vi "Lookup Group.vi"(7 "Group Type (Abstract)":refnum<class "GroupAbstract.lvclass">, 8 "error in (no error)":errorcluster, 10 "Group Name":string, 11 "Module in":refnum<class "Module.lvclass">) -> (0 "error out":errorcluster, 2 "Group":refnum<class "GroupAbstract.lvclass">, 3 "Module out":refnum<class "Module.lvclass">)   [LabVIEW 2020, in "Volatus.lvlib" / "Module.lvclass"]
uses:
  Module.lvclass
  Module.lvclass/Module.ctl
  VolatusAPI/VolatusAPI.lvclass
  lv-vecto/Vecto/GroupAbstract/GroupAbstract.lvclass
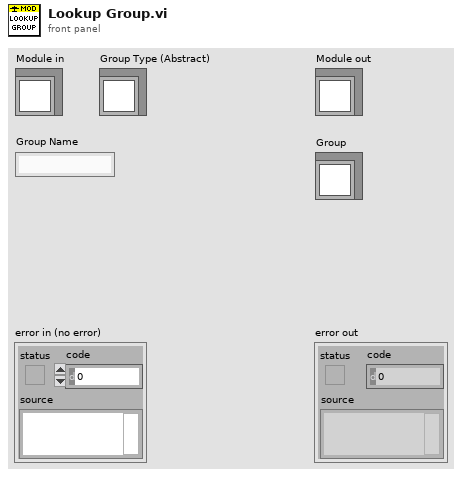
[diagram p1: front panel]
types:
  T1 = map{string, refnum<class "GroupAbstract.lvclass">}
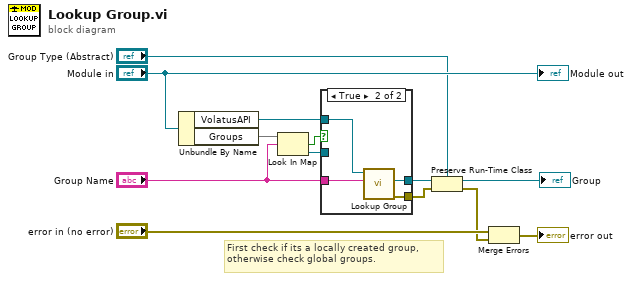
[diagram p0: block diagram]
diagram:
  # "First check if its a locally created group, otherwise check global groups."
  n1 = Unbundle By Name("Module in") -> ("VolatusAPI"=w8:refnum<class "VolatusAPI.lvclass">, "Groups"=w11:T1)
  n2 = Look In Map(map=w11, key="Group Name") -> (key not found?=w10:bool, value=w9:refnum<class "GroupAbstract.lvclass">)  [unwired: 1 in]
  n3 = case shown="True" w10 {
    tunnel: w9 -> [w14 _]
    tunnel: w8 -> [_ w18]
    tunnel: "Group Name" -> [_ w17]
    tunnel: [w14 w16] -> w6
    tunnel: [_ w15] -> w4
    frame False {
    }
    frame True {
      n4 = call "Lookup Group.vi"("Group Name"=w17, "VolatusAPI in"=w18) -> ("error out"=w15:errorcluster, "Group"=w16:refnum<class "GroupAbstract.lvclass">)  [unwired: 7 in, 1 out]
    }
  }
  n5 = Preserve Run-Time Class(object in=w6, error in=w4, 2:"Group Type (Abstract)") -> (object out=→"Group":refnum<class "GroupAbstract.lvclass">, error out=w1:errorcluster)
  n6 = Merge Errors("error in (no error)", w1) -> (→"error out":errorcluster)
  "Module out" <- "Module in"
